vi "Server pre-Build Action.vi"(6 "Top Level/Always Included VIs":path[](array[path]), 7 "Main Destination Path":path, 9 "Target Name":string, 10 "Build Specification Name":string, 11 "Project Path":path) -> (0 "error out":errorcluster)   [LabVIEW 2020]
doc: "This is called before build of TWM client and it sets build version to version holding VI. This is necessary to ensure version compatibility checking between TWM and TWM client."
uses:
  23065927-9aa0-479e-a8f7-bdd98458ad32.vi
  <vilib>/AppBuilder/AB_API_Simple/Set Build Specification Version (path).vi
  <vilib>/AppBuilder/AB_API_Simple/Get Build Specification Version (path).vi
  TWM client/TWM Client Version.vi
  <vilib>/Comparison/Equal/Equal Functor/Equal Functor.lvclass
  <vilib>/AppBuilder/AB_API_Simple/NI_App_Builder_API.lvlib
  TWM client/TWM Client.lvlib
panel:
  in  "btn ok":bool
  in  "ref builds":i32(listbox) caption="Select reference build for which the TWM client will be built:"
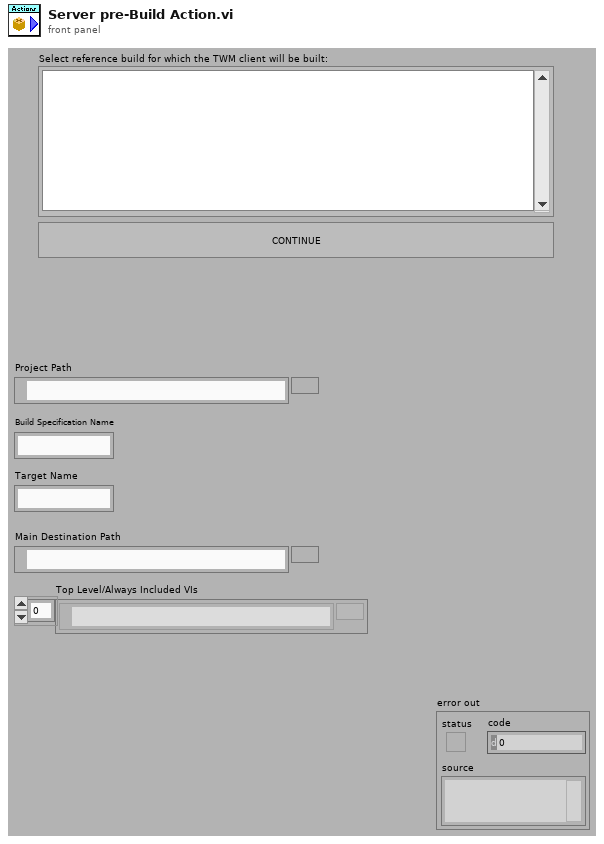
[diagram p1: front panel]
types:
  T1 = typedef "NI_App_Builder_API.lvlib/Build Specification Version.ctl" = cluster{"Major":u16, "Minor":u16, "Fix":u16, "Build":u16}
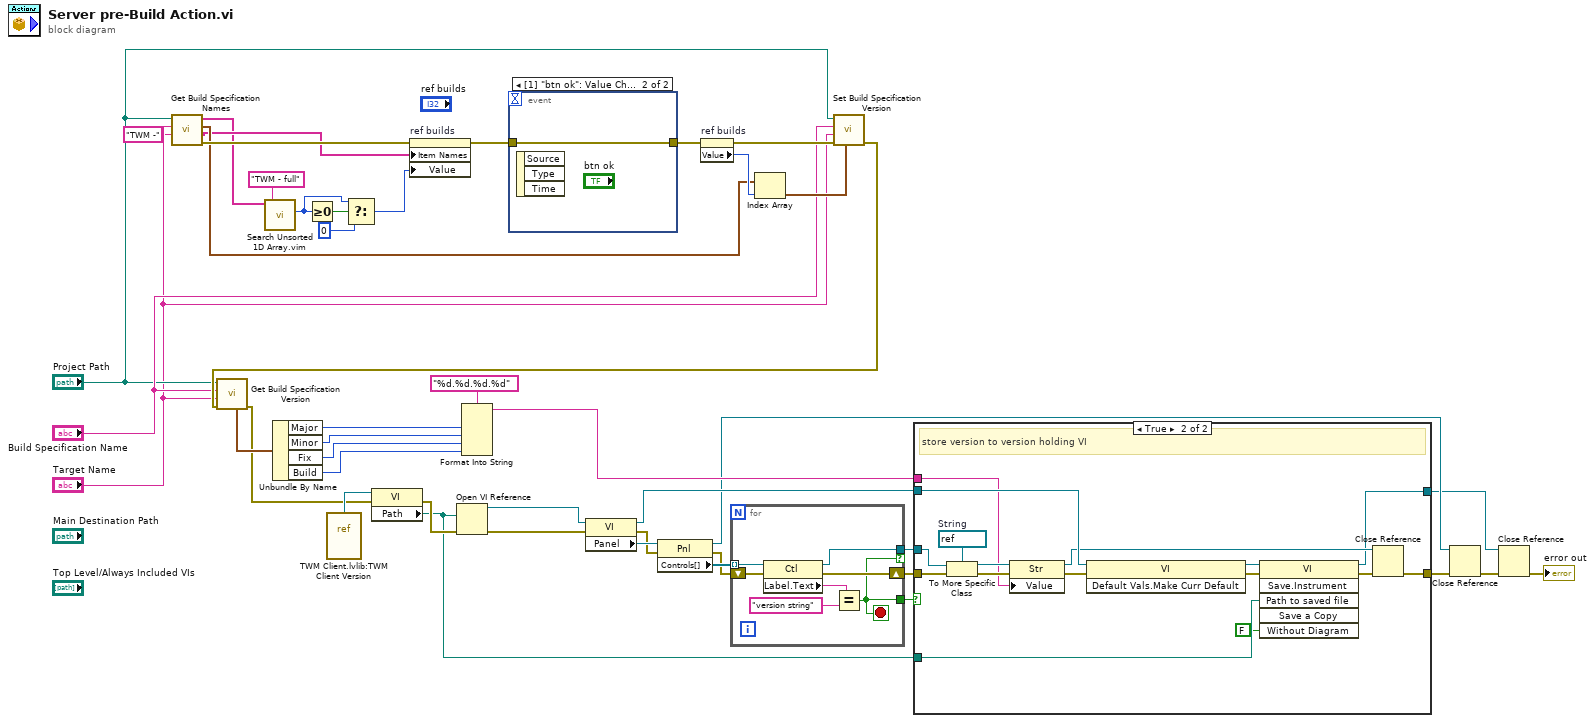
[diagram p0: block diagram]
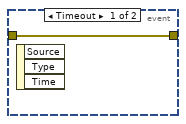
[diagram p2: hidden frame]
diagram:
  n1 = call "Get Build Specification Names.vi"("Build specification regexp filter (.*)"="TWM -", "Target Name"="Target Name", "Project Path"="Project Path") -> ("error out"=w11:errorcluster, "Build specification names with version string"=w9:string[], "Build spec vections"=w10:T1[], "Build specification names"=w8:string[])  [unwired: 4 in, 1 out]
  n2 = call "Search Unsorted 1D Array.vim"("element"="TWM - full" ("format string"), "unsorted 1D array"=w8) -> ("index of element"=w21:i32)  [unwired: 9 in]
  n3 = Greater Or Equal To 0?(x=w21) -> (x >= 0?=w22:bool)
  n4 = vi-ref "TWM Client.lvlib:TWM Client Version.vi"() -> (w4:refnum<vi>)
  n5 = Select(t=w21, s=w22, f=0) -> (s? t:f=w19:i32)
  n6 = property on="ref builds" class="LstBox (strict)"(error in=w11, "Item Names"=w9, "Value"=w19) -> (error out=w18:errorcluster)  [unwired: 1 in, 1 out]
  n7 = event shown="[1] \"btn ok\": Value Change;  Panel Close" {
    selector: _ -> [_ _]
    dyn-events: _ -> [_ _]
    timeout: _ -> [_ _]
    tunnel: w18 -> [w46 w47]
    tunnel: [w46 w47] -> w16
    event Timeout {
      n8 = event-data() -> ()  [unwired: 1 in, 3 out]
    }
    event "btn ok": Value Change; Panel Close {
      n9 = event-data() -> ()  [unwired: 1 in, 3 out]
    }
  }
  n10 = property on="ref builds" class="LstBox (strict)"(error in=w16) -> (error out=w14:errorcluster, "Value"=w13:i32)  [unwired: 1 in, 1 out]
  n11 = Index Array(array=w10, index=w13) -> (element=w15:T1)
  n12 = call-poly <vilib>:"Set Build Specification Version.vi"("Build Specification Version"=w15, "error in (no error)"=w14, "Name of target (My Computer)"="Target Name", "Name of build specification"="Build Specification Name", "Path to project"="Project Path") -> ("error out"=w17:errorcluster)  [unwired: 6 in]
  n13 = call-poly <vilib>:"Get Build Specification Version.vi"("error in (no error)"=w17, "Name of target (My Computer)"="Target Name", "Name of build specification"="Build Specification Name", "Path to project"="Project Path") -> ("error out"=w2:errorcluster, "Build Specification Version"=w45:T1)  [unwired: 6 in]
  n14 = Unbundle By Name(w45) -> ("Major"=w43:u16, "Minor"=w42:u16, "Fix"=w41:u16, "Build"=w40:u16)
  n15 = property class="VI"(reference=w4, error in=w2) -> (error out=w3:errorcluster, "Path"=w1:path)  [unwired: 1 out]
  n16 = Open VI Reference(vi path=w1, error in (no error)=w3) -> (vi reference=w29:refnum<vi>, error out=w30:errorcluster)  [unwired: 4 in]
  n17 = Format Into String(format string="%d.%d.%d.%d", w43, w42, w41, w40) -> (resulting string=w32:string)  [unwired: 2 in, 1 out]
  n18 = property class="VI"(reference=w29, error in=w30) -> (reference out=w31:refnum<vi>, error out=w37:errorcluster, "Panel"=w39:refnum<vi>)
  n19 = property class="Pnl"(reference=w39, error in=w37) -> (reference out=w27:refnum<vi>, error out=w36:errorcluster, "Controls[]"=w38:refnum<vi>[])
  n20 = for {
    tunnel: w38 -> [w54] mode=indexing
    shift-right: [w52] -> w34
    shift-left: w36 -> [w53]
    tunnel: [w49] -> w33 if=w48
    tunnel: [w48] -> w35
    stop <- w48 stop-if-true
    n21 = property class="Ctl"(reference=w54, error in=w53) -> (reference out=w49:refnum<vi>, error out=w52:errorcluster, "Label.Text"=w51:string)
    n22 = Equal?(x=w51, y="version string") -> (x = y?=w48:bool)
  }
  n23 = case shown="True" w35 {
    tunnel: w34 -> [w56 w72]
    tunnel: w33 -> [_ w70]
    tunnel: w32 -> [_ w64]
    tunnel: w31 -> [w55 w67]
    tunnel: [w56 w60] -> w28
    tunnel: [w55 w59] -> w25
    tunnel: w1 -> [_ w58]
    frame False {
    }
    frame True {
      w71 = refnum<vi> refnum  # String
      # "store version to version holding VI"
      n24 = To More Specific Class(target class=w71, reference=w70, error in=w72) -> (specific class reference=w68:refnum<vi>, error out=w69:errorcluster)
      n25 = property class="Str"(reference=w68, error in=w69, "Value"=w64) -> (reference out=w61:refnum<vi>, error out=w63:errorcluster)
      n26 = invoke class="VI" method="Default Vals.Make Curr Default"(reference=w67, error in=w63) -> (reference out=w66:refnum<vi>, error out=w65:errorcluster)  [unwired: 1 in, 1 out]
      n27 = invoke class="VI" method="Save.Instrument"(reference=w66, error in=w65, "Path to saved file"=w58, "Without Diagram"=FALSE) -> (reference out=w59:refnum<vi>, error out=w62:errorcluster)  [unwired: 2 in, 4 out]
      n28 = Close Reference(reference=w61, error in (no error)=w62) -> (error out=w60:errorcluster)
    }
  }
  n29 = Close Reference(reference=w27, error in (no error)=w28) -> (error out=w26:errorcluster)
  n30 = Close Reference(reference=w25, error in (no error)=w26) -> (error out=→"error out":errorcluster)
